vi "WPI_DMAOpen.vi"   [LabVIEW 2017]
doc: "Opens a reference to the DMA stream from the FPGA of the roboRIO. You must open a reference before using any other VIs on this palette. You can have only one DMA stream open at a time. If you want to open a new DMA stream, use the Close VI to close the reference to the current DMA stream first.\n\nThis software is licensed. Open the labview\\readme\\WPI Robotics Library Open Source License.txt file for more information."
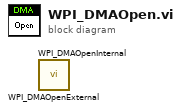
[diagram p0: block diagram]
diagram:
  n1 = call <vilib>:"WPI_DMAOpenExternal.vi"() -> ()  [unwired: 10 in, 2 out]
  n2 = call <vilib>:"WPI_DMAOpenInternal.vi"() -> ()  [unwired: 10 in, 2 out]
